vi "DIO_WriteAll.vi"(7 "DeviceIndex":i32 max=32, 8 "error in (no error)":errorcluster, 10 "OutBytes":T1 {"Out Byte 3" format="%08b"; "Out Byte 2" format="%08b"; "Out Byte 1" format="%08b"; "Out Byte 0" format="%08b"}) -> (0 "error out":errorcluster)   [LabVIEW 2012]
doc: "This VI can be used to set all the bits that are configured as outputs."
uses:
  Controls/DIO_bytemask.ctl
  Windows/System32/AIOUSB.dll
panel:
  out "Return Value":u32
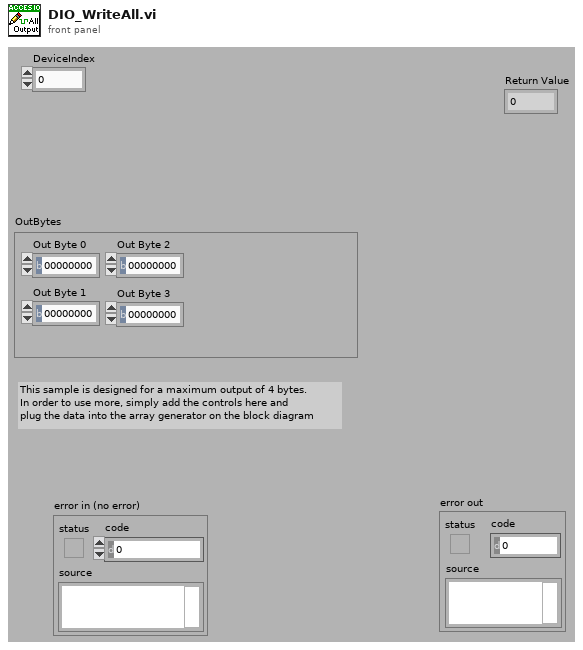
[diagram p1: front panel]
types:
  T1 = typedef "DIO_bytemask.ctl" = cluster{"Out Byte 0":u8, "Out Byte 1":u8, "Out Byte 2":u8, "Out Byte 3":u8}
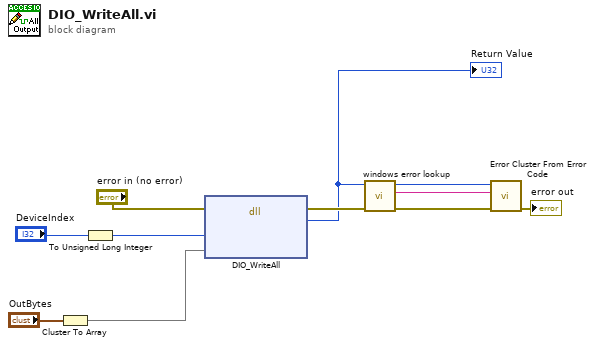
[diagram p0: block diagram]
diagram:
  n1 = Cluster To Array(cluster="OutBytes") -> (array=w8:u8[])
  n2 = To Unsigned Long Integer(number="DeviceIndex") -> (unsigned 32bit integer=w1:u32)
  n3 = dll-call lib="C:/Windows/System32/AIOUSB.dll" fn="DIO_WriteAll"(error in="error in (no error)", "DeviceIndex"=w1, "pData"=w8) -> (error out=w3:errorcluster, "return type"=w2:u32)  [unwired: 4 in, 1 out]
  "Return Value" <- w2
  n4 = call "windows error lookup.vi"("error in (no error)"=w3, "Error Code"=w2) -> ("error out"=w4:errorcluster, "error message (\"\")"=w6:string)  [unwired: 8 in]
  n5 = call <vilib>:"Error Cluster From Error Code.vi"("error in (no error)"=w4, "error message (\"\")"=w6, "error code (0)"=w2) -> ("error out"=→"error out":errorcluster)  [unwired: 6 in]
